vi "Update Status.vi"(8 "error in (no error)":errorcluster, 10 "Status":string, 11 "Person In":refnum<class "Person.lvclass">) -> (0 "error out":errorcluster, 3 "Person Out":refnum<class "Person.lvclass">)   [LabVIEW 2021, in "Person.lvclass"]
uses:
  Person.lvclass
  C:/Program Files (x86)/National Instruments/LabVIEW 2021/vi.lib/Astemes/Triarc Framework/Process/Process.lvclass
  <vilib>/Astemes/Triarc Framework/Process/Process.lvclass/Process.ctl
  Person.lvclass/Person.ctl
  <vilib>/Utility/error.llb/Clear Errors.vi
  <vilib>/Astemes/Triarc Framework/Process/Private/SubVIs/Handle Debug Data.vi
  <vilib>/Utility/High Resolution Relative Seconds.vi
  <vilib>/Utility/error.llb/Error Cluster From Error Code.vi
  C:/Program Files (x86)/National Instruments/LabVIEW 2021/vi.lib/Astemes/Triarc Framework/View/View.lvclass
  C:/Program Files (x86)/National Instruments/LabVIEW 2021/vi.lib/Astemes/Triarc Framework/Base/Base.lvclass
  C:/Program Files (x86)/National Instruments/LabVIEW 2021/vi.lib/Astemes/Triarc Framework/Error Handler Interface/Error Handler Interface.lvclass
  C:/Program Files (x86)/National Instruments/LabVIEW 2021/vi.lib/Astemes/Triarc Framework/Logging/Logging.lvclass
  C:/Git/astemes-triarc-examples/Coffee Shop/Processes/People/Person/Person.lvclass
  <vilib>/Astemes/Triarc Framework/Process/Process.lvclass
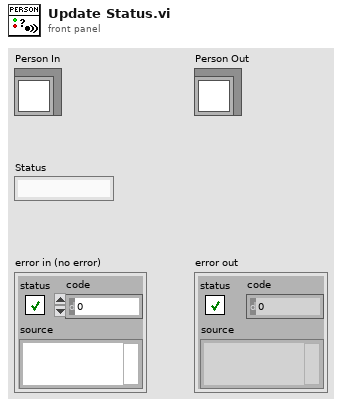
[diagram p1: front panel]
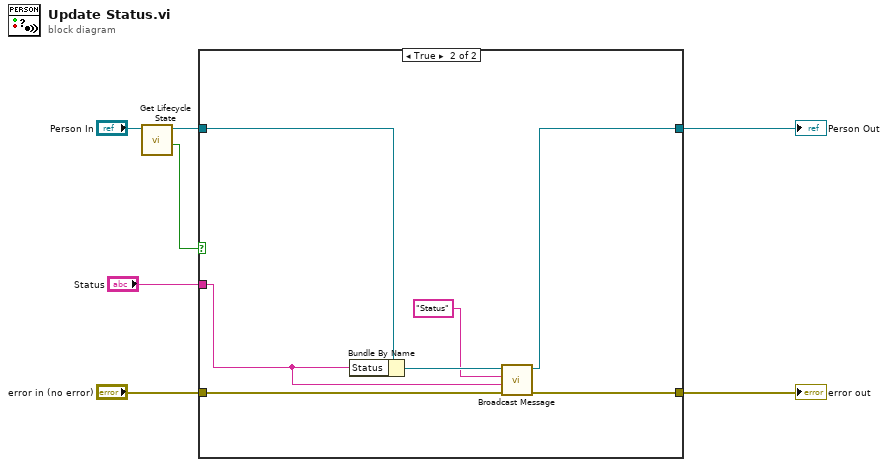
[diagram p0: block diagram]
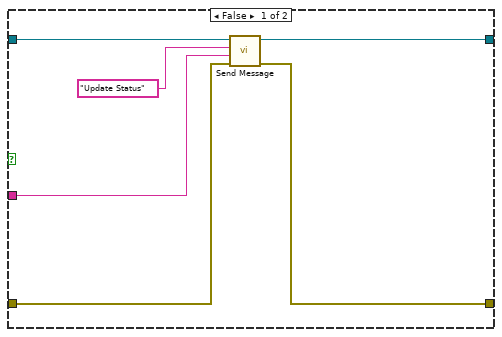
[diagram p2: hidden frame]
diagram:
  n1 = call <vilib>:"Get Lifecycle State.vi"("Process In"="Person In") -> ("In Process Loop?"=w1:bool, "Process Out"=w2:refnum<class "Person.lvclass">)  [unwired: 7 in, 2 out]
  n2 = case shown="True" w1 {
    tunnel: "error in (no error)" -> [w13 w18]
    tunnel: [w12 w17] -> w6
    tunnel: w2 -> [w11 w19]
    tunnel: [w10 w16] -> w4
    tunnel: "Status" -> [w8 w15]
    frame False {
      n3 = call <vilib>:"Send Message.vi"("error in (no error)"=w13, "Message Data"=w8, "Message"="Update Status", "Process In"=w11) -> ("error out"=w12:errorcluster, "Process Out"=w10:refnum<class "Person.lvclass">)  [unwired: 6 in]
    }
    frame True {
      n4 = Bundle By Name(cluster=w19, "Status"=w15) -> (w20:refnum<class "Person.lvclass">)
      n5 = call-dynamic "Broadcast Message.vi"("error in (no error)"=w18, "Message Data"=w15, "Message"="Status", "Process In"=w20) -> ("error out"=w17:errorcluster, "Process Out"=w16:refnum<class "Person.lvclass">)  [unwired: 6 in]
    }
  }
  "error out" <- w6
  "Person Out" <- w4
